vi "数值转换.vi"(8 "error in (no error)":errorcluster caption="错误输入（无错误）", 11 "Digital Waveform":digitalwaveform(waveform)) -> (0 "error out":errorcluster caption="错误输出", 3 "Waveform":waveform(dbl))   [LabVIEW 2019]
uses:
  <vilib>/Waveform/DWDTOps.llb/DWDT Digital to Binary U8.vi
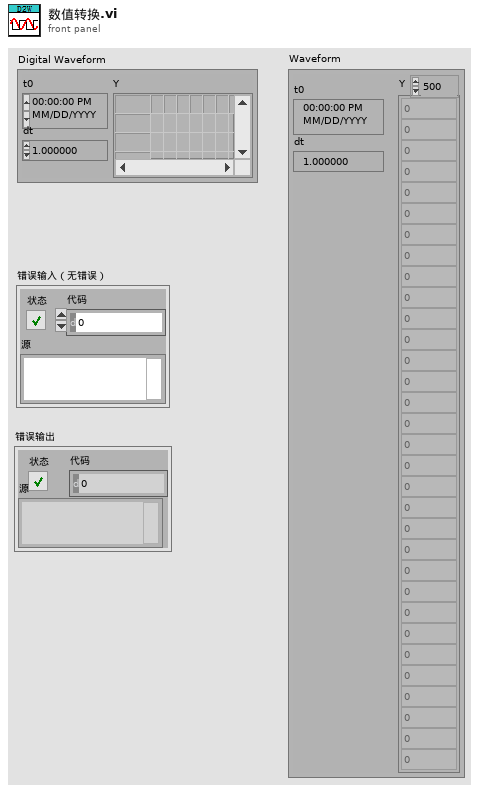
[diagram p1: front panel]
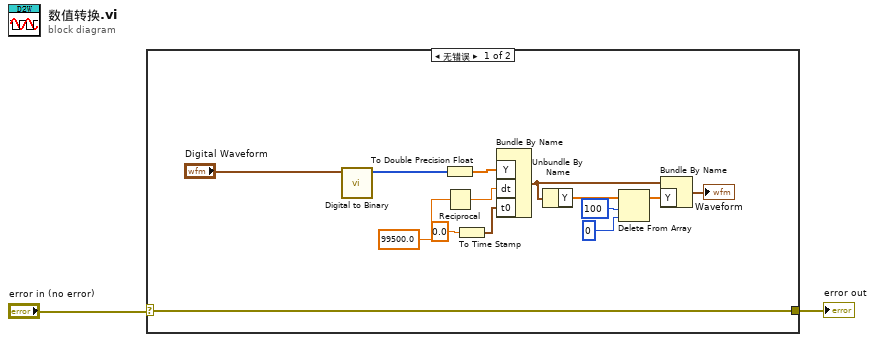
[diagram p0: block diagram]
diagram:
  n1 = case shown="无错误" "error in (no error)" {
    selector: "error in (no error)" -> [w3 w17]
    tunnel: [w3 w17] -> w1
    frame No Error {
      n2 = call-poly <vilib>:"Digital to Binary.vi"("digital waveform"="Digital Waveform") -> ("binary array"=w4:u8[])  [unwired: 9 in, 1 out]
      n3 = To Double Precision Float(number=w4) -> (double precision float=w8:dbl[])
      n4 = Reciprocal(x=99500.0) -> (1/x=w10:dbl)
      n5 = To Time Stamp(1:0.0 ("数字")) -> (0:w6:timestamp)
      n6 = Bundle By Name("Y"=w8, "dt"=w10, "t0"=w6) -> (w9:waveform(dbl))  [unwired: 1 in]
      n7 = Unbundle By Name(w9) -> ("Y"=w11:dbl[])
      n8 = Delete From Array(array=w11, length=100 ("长度"), index=0 ("索引")) -> (array with subset deleted=w14:dbl[])  [unwired: 1 out]
      n9 = Bundle By Name(cluster=w9, "Y"=w14) -> (→"Waveform":waveform(dbl))
    }
    frame Error {
    }
  }
  "error out" <- w1
